vi "Get Dependent File Properties.vi"(8 "error in (no error)":errorcluster, 10 "property names":string[](array[string]), 11 "Device Ref in":T5 format="%.0x") -> (0 "error out":errorcluster, 2 "property values":T1[](array[typedef]), 3 "Device Ref out":T5 format="%.0x")   [LabVIEW 2019, in "SEECD System Explorer.lvlib"]
uses:
  <vilib>/NI VeriStand/Custom Device API/Custom Device Item Ref.ctl
  <vilib>/NI VeriStand/Custom Device API/Custom Device File Dependency.ctl
  <vilib>/NI VeriStand/Custom Device API/Path Specification.ctl
  <vilib>/NI VeriStand/Custom Device API/Path Type.ctl
  <vilib>/NI VeriStand/Custom Device API/Custom Device Supported Target.ctl
  NationalInstruments.VeriStand.SystemDefinitionAPI
  NationalInstruments.VeriStand.SystemStorage
  SEECD System Explorer.lvlib
  <vilib>/NI VeriStand/Custom Device API/Custom Device API.lvlib
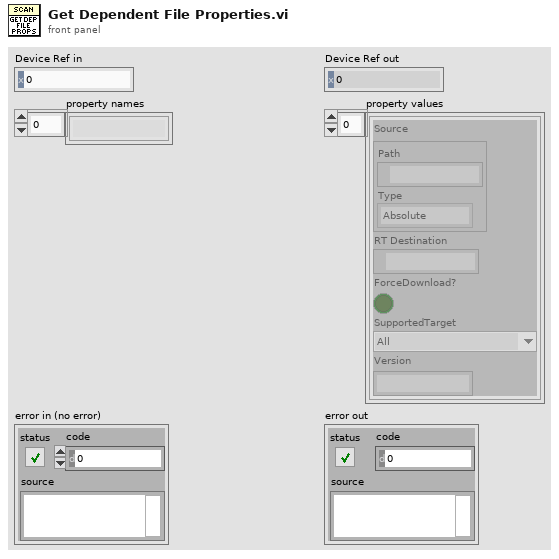
[diagram p1: front panel]
types:
  T1 = typedef "Custom Device API.lvlib/Custom Device File Dependency.ctl" = cluster{"Source":T2, "RT Destination":path, "ForceDownload?":bool, "SupportedTarget":T4, "Version":string}
  T2 = typedef "Custom Device API.lvlib/Path Specification.ctl" = cluster{"Path":path, "Type":T3}
  T3 = typedef "Custom Device API.lvlib/Path Type.ctl" = enum16{"Absolute", "To Base", "To Common Data Dir", "To Application Data Dir"}
  T4 = typedef "Custom Device API.lvlib/Custom Device Supported Target.ctl" = enum16{"All", "PharLap", "VxWorks", "Windows", "Linux_32_ARM", "Linux_x64", "PharLap & Windows", "PharLap & VxWorks", "VxWorks & Windows"}
  T5 = typedef "Custom Device API.lvlib/Custom Device Item Ref.ctl" = u64
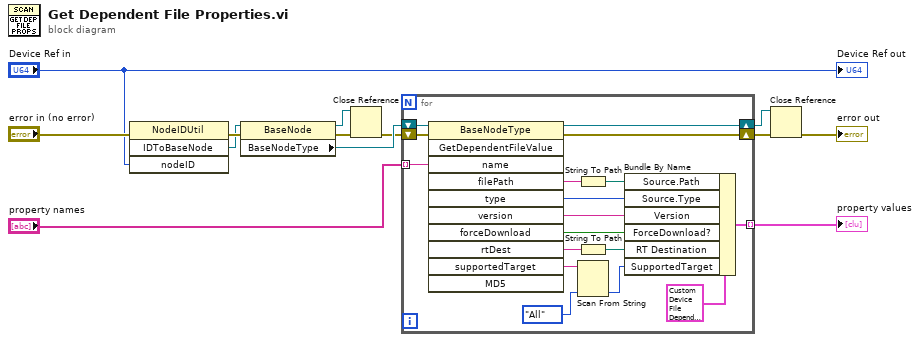
[diagram p0: block diagram]
diagram:
  n1 = invoke class="NodeIDUtil" method="IDToBaseNode"(error in="error in (no error)", "nodeID"="Device Ref in") -> (error out=w11:errorcluster, "IDToBaseNode"=w10:refnum<k24>)  [unwired: 2 in, 2 out]
  n2 = property class="BaseNode"(reference=w10, error in=w11) -> (reference out=w8:refnum<k24>, error out=w13:errorcluster, "BaseNodeType"=w6:refnum<k24>)
  n3 = Close Reference(reference=w8, error in (no error)=w13) -> (error out=w5:errorcluster)
  n4 = for {
    tunnel: [w28] -> w9 mode=indexing
    tunnel: "property names" -> [w18] mode=indexing
    shift-right: [w16] -> w3
    shift-left: w6 -> [w19]
    shift-right: [w15] -> w4
    shift-left: w5 -> [w17]
    n5 = invoke class="BaseNodeType" method="GetDependentFileValue"(reference=w19, error in=w17, "name"=w18) -> (reference out=w16:refnum<k24>, error out=w15:errorcluster, "filePath"=w26:string, "type"=w25:i32, "version"=w20:string, "forceDownload"=w24:bool, "rtDest"=w23:string, "supportedTarget"=w22:string)  [unwired: 8 in, 3 out]
    n6 = String To Path(string=w26) -> (path=w30:path)
    n7 = String To Path(string=w23) -> (path=w21:path)
    n8 = Scan From String(input string=w22, default 1=Custom_Device_Supported_Target."All" ("SupportedTarget")) -> (output 1=w29:T4)  [unwired: 3 in, 3 out]
    n9 = Bundle By Name(cluster=T1 {"Source"={"Path"=path "", "Type"=enum."Absolute"}, "RT Destination"=path "", "ForceDownload?"=FALSE, "SupportedTarget"=enum."PharLap", "Version"=""} ("Dependency"), "Source.Path"=w30, "Source.Type"=w25, "Version"=w20, "ForceDownload?"=w24, "RT Destination"=w21, "SupportedTarget"=w29) -> (w28:T1)
  }
  "property values" <- w9
  n10 = Close Reference(reference=w3, error in (no error)=w4) -> (error out=→"error out":errorcluster)
  "Device Ref out" <- "Device Ref in"
